vi "intiStimulus.vi"(6 "index":i32, 8 "error in (no error)":errorcluster, 9 "Params":T1={"Mice ID"=[], "ExpType"=[], "Trial Interval"=[], "Pulse Duration"=[158.0, 152.0, 156.0, 167.0, 172.0], "microL_per_pulse"=[6.0, 6.0, 6.0, 6.0, 6.0], "Response Interval"=[1000.0, 1000.0, 1000.0, 1000.0, 1000.0], "Bad Delay"=[], "Response Period"=[], "liquid_type"="water", "Stimuli"=[], "Rewarded Stimuli"=[], "AirDur"=[]} {"AirDur" format="%#_13g"}, 10 "Monitor parameters":dbl[][](array[numeric])=[[100.0, 100.0, 0.0, 0.0], [100.0, 100.0, 100.0, 0.0], [100.0, 100.0, 200.0, 0.0], [100.0, 100.0, 300.0, 0.0], [100.0, 100.0, 400.0, 0.0]], 11 "Stimulus in":refnum<class "Stimulus.lvclass">) -> (0 "error out":errorcluster, 3 "Stimulus out":refnum<class "Stimulus.lvclass">)   [LabVIEW 2014, in "Stimulus.lvclass"]
uses:
  Stimulus.lvclass
  ParamsArray.ctl
  Stimulus.lvclass/Stimulus.ctl
  <vilib>/regexp/Match Regular Expression.xnode
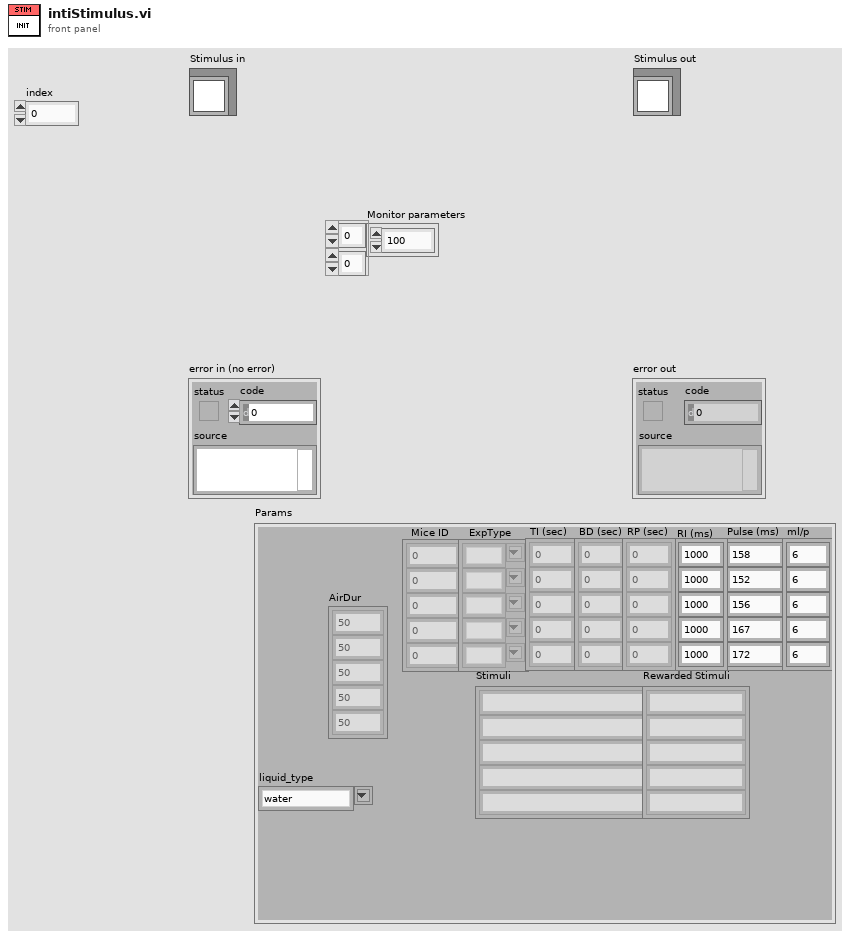
[diagram p1: front panel]
types:
  T1 = typedef "ParamsArray.ctl" = cluster{"Mice ID":dbl[], "ExpType":string[], "Trial Interval":dbl[], "Pulse Duration":dbl[], "microL_per_pulse":dbl[], "Response Interval":dbl[], "Bad Delay":dbl[], "Response Period":dbl[], "liquid_type":string, "Stimuli":string[], "Rewarded Stimuli":string[], "AirDur":dbl[]}
  T2 = typedef "IMAQ Image.ctl" = refnum<image>
  T3 = typedef "ParamsArray2.ctl" = cluster{"liquid_type":string, "Mouse ID":dbl, "Trial Interval":dbl, "Pulse Duration":dbl, "microL_per_pulse":dbl, "Response Interval":dbl, "Bad Delay":dbl, "Response Period":dbl, "Stimuli":string, "Rewarded Stimuli":string, "Air Dur":dbl, "ExpType":string}
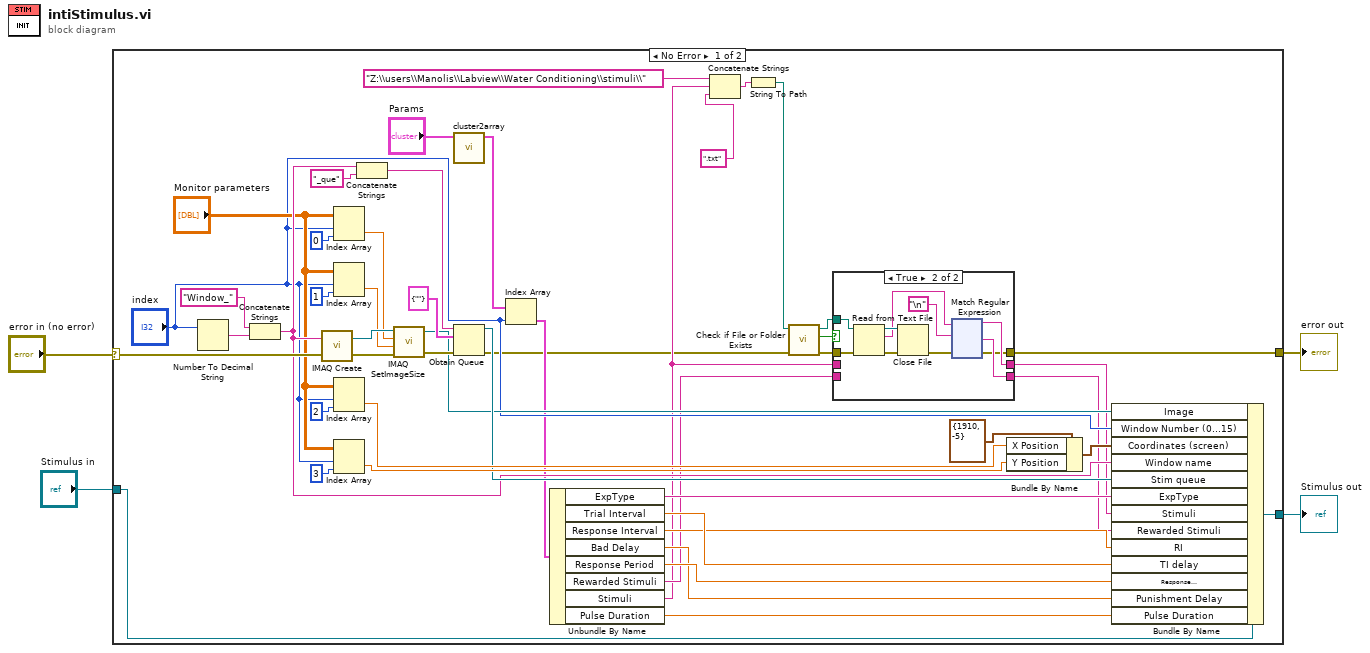
[diagram p0: block diagram]
diagram:
  n1 = case shown="No Error" "error in (no error)" {
    selector: "error in (no error)" -> [w52 w180]
    tunnel: [w6 w180] -> w1
    tunnel: [w33 w181] -> w2
    tunnel: "Stimulus in" -> [w34 w181]
    frame No Error {
      n2 = Number To Decimal String(number="index") -> (decimal integer string=w43:string)  [unwired: 1 in]
      n3 = Concatenate Strings("Window_", w43) -> (w38:string)
      n4 = call "IMAQ Create"("Image Name"=w38, "error in (no error)"=w52) -> ("New Image"=w50:T2, "error out"=w51:errorcluster)  [unwired: 3 in]
      n5 = Index Array(array="Monitor parameters", index (row)="index", index (col)=0 ("disabled index (col)")) -> (element=w49:dbl)
      n6 = Index Array(array="Monitor parameters", index (row)="index", index (col)=1 ("disabled index (col)")) -> (element=w48:dbl)
      n7 = Index Array(array="Monitor parameters", index (row)="index", index (col)=2 ("disabled index (col)")) -> (element=w46:dbl)
      n8 = Index Array(array="Monitor parameters", index (row)="index", index (col)=3 ("disabled index (col)")) -> (element=w45:dbl)
      n9 = Concatenate Strings(w38, "_que" ("string")) -> (w36:string)
      n10 = call "IMAQ SetImageSize"("error in (no error)"=w51, "Y Resolution"=w48, "X Resolution"=w49, "Image"=w50) -> ("error out"=w41:errorcluster, "Image Out"=w35:T2)  [unwired: 1 in]
      n11 = call "cluster2array.vi"("Params"="Params") -> ("Array"=w26:T3[])  [unwired: 10 in]
      n12 = Obtain Queue(name (unnamed)=w36, element data type=cluster{"Stim":string} {"Stim"=""} ("Stim element"), error in (no error)=w41) -> (queue out=w39:refnum<queue>, error out=w8:errorcluster)  [unwired: 2 in, 1 out]
      n13 = Index Array(array=w26, index="index") -> (element=w24:T3)
      n14 = Unbundle By Name(w24) -> ("ExpType"=w23:string, "Trial Interval"=w22:dbl, "Response Interval"=w21:dbl, "Bad Delay"=w19:dbl, "Response Period"=w20:dbl, "Rewarded Stimuli"=w17:string, "Stimuli"=w9:string, "Pulse Duration"=w18:dbl)
      n15 = Concatenate Strings("Z:\\users\\Manolis\\Labview\\Water Conditioning\\stimuli\\", w9, ".txt") -> (w13:string)
      n16 = String To Path(string=w13) -> (path=w14:path)
      n17 = call <vilib>:"Check if File or Folder Exists.vi"("error in (no error)"=w8, "path"=w14) -> ("error out"=w7:errorcluster, "file or folder exists?"=w11:bool, "dup path"=w10:path)  [unwired: 7 in]
      n18 = case shown="True" w11 {
        tunnel: w9 -> [w54 _]
        tunnel: w17 -> [w55 _]
        tunnel: [w55 w60] -> w16
        tunnel: [w54 w61] -> w15
        tunnel: w10 -> [_ w64]
        tunnel: w7 -> [w53 w57]
        tunnel: [w53 w56] -> w6
        frame False {
        }
        frame True {
          n19 = Read from Text File(file (use dialog)=w64, error in=w57) -> (refnum out=w65:refnum<file>, text=w62:string, error out=w59:errorcluster)  [unwired: 2 in, 1 out]
          n20 = Close File(refnum=w65, error in=w59) -> (error out=w58:errorcluster)  [unwired: 1 out]
          n21 = xnode "Match Regular Expression"("input string"=w62, "regular expression"="\n", "error in"=w58) -> ("before match"=w61:string, "after match"=w60:string, "error out"=w56:errorcluster)  [unwired: 3 in, 2 out]
        }
      }
      n22 = Bundle By Name(cluster=cluster{"X Position":i32, "Y Position":i32} {"X Position"=1910, "Y Position"=-5} ("Coordinates (screen)"), "X Position"=w46, "Y Position"=w45) -> (w42:cluster{"X Position":i32, "Y Position":i32})
      n23 = Bundle By Name(cluster=w34, "Image"=w35, "Window Number (0...15)"="index", "Coordinates (screen)"=w42, "Window name"=w38, "Stim queue"=w39, "ExpType"=w23, "Stimuli"=w15, "Rewarded Stimuli"=w16, "RI"=w21, "TI delay"=w22, "Response \nperiod"=w20, "Punishment Delay"=w19, "Pulse Duration"=w18) -> (w33:refnum<class "Stimulus.lvclass">)
    }
    frame Error {
    }
  }
  "error out" <- w1
  "Stimulus out" <- w2
